vi "Register Loader.vi"(6 "timeout (ms)":i32=5000, 8 "error in":errorcluster, 10 "Loader Info":T1, 11 "gRPC ID in":T3) -> (0 "error out":errorcluster, 3 "gRPC ID out":T3)   [LabVIEW 2021, in "CIFManagerClientWrapper.lvlib"]
uses:
  CIFManagerClientWrapper.lvlib
  <vilib>/gRPC/LabVIEW gRPC Library/Shared/grpcId.ctl
  CIF_Manager_client/RPC Messages/cif_management_common_LoaderInfoFull.ctl
  CIF_Manager_client/RPC Messages/cif_management_common_LoaderType.ctl
  CIF_Manager_client/RPC Messages/cif_manager_RegisterPluginLoaderRequest.ctl
  CIF_Manager_client/CIF_Manager_client.lvlib
  <vilib>/gRPC/LabVIEW gRPC Library/grpc-lvsupport-release.lvlib
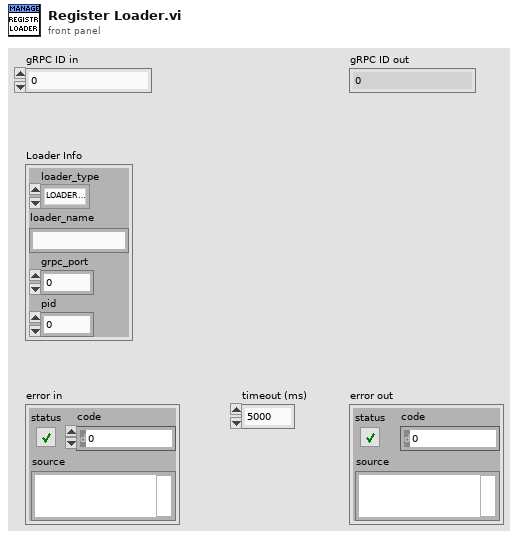
[diagram p1: front panel]
types:
  T1 = typedef "CIF_Manager_client.lvlib/cif_management_common_LoaderInfoFull.ctl" = cluster{"loader_type":T2, "loader_name":string, "grpc_port":i32, "pid":u32}
  T2 = typedef "CIF_Manager_client.lvlib/cif_management_common_LoaderType.ctl" = enum32{"LOADERTYPE_UNKNOWN", "LOADERTYPE_LABVIEW"}
  T3 = typedef "grpc-lvsupport-release.lvlib/grpcId.ctl" = u64
  T4 = typedef "CIF_Manager_client.lvlib/cif_manager_RegisterPluginLoaderRequest.ctl" = cluster{"loader_info":T1}
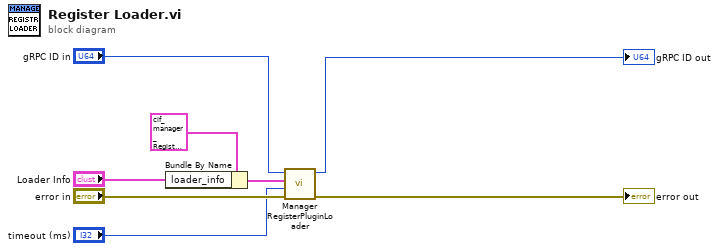
[diagram p0: block diagram]
diagram:
  n1 = Bundle By Name(cluster=T4 {"loader_info"={"loader_type"=enum."LOADERTYPE_UNKNOWN", "loader_name"="", "grpc_port"=0, "pid"=0}} ("Request Data"), "loader_info"="Loader Info") -> (w1:T4)
  n2 = call "Manager RegisterPluginLoader.vi"("error in"="error in", "timeout (ms)"="timeout (ms)", "Request Data"=w1, "gRPC ID"="gRPC ID in") -> ("error out"=→"error out":errorcluster, "gRPC ID out"=→"gRPC ID out":T3)  [unwired: 5 in, 1 out]
